vi "Read.vi"(7 "timeout (100ms)":i32=100, 8 "error in (no error)":errorcluster, 9 "Interlock in":bool, 11 "Interlock in":refnum<class "Interlock.lvclass">) -> (0 "error out":errorcluster, 1 "Interlock out":bool, 2 "Data out":variant, 3 "Interlock out":refnum<class "Interlock.lvclass">, 4 "IL Action":refnum<class "IL Action.lvclass">[](array[class]))   [LabVIEW 2015, in "Interlocks.lvlib" / "Interlock.lvclass"]
uses:
  Interlock.lvclass
  IL Action/IL Action.lvclass
  Interlock.lvclass/Interlock.ctl
  State Enum.ctl
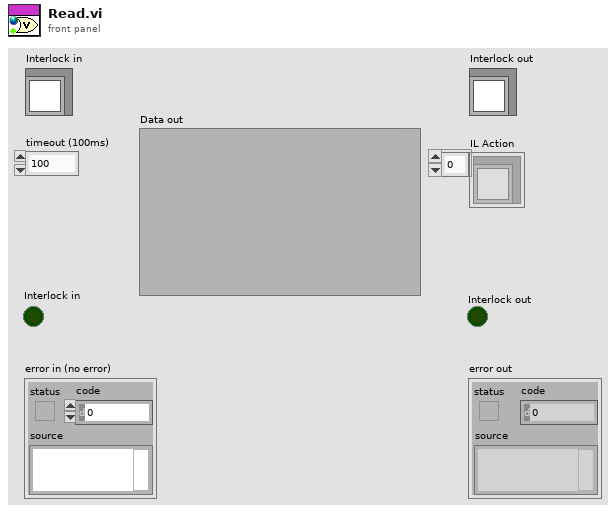
[diagram p1: front panel]
types:
  T1 = typedef "Interlocks.lvlib/Interlock.lvclass/State Enum.ctl" = enum16{"Ok", "Error", "Interlock", "Out of Range", "Is ON", "Is OFF", "Denied", "Not Allowed", "Sample Allow", "Sample Deny"}
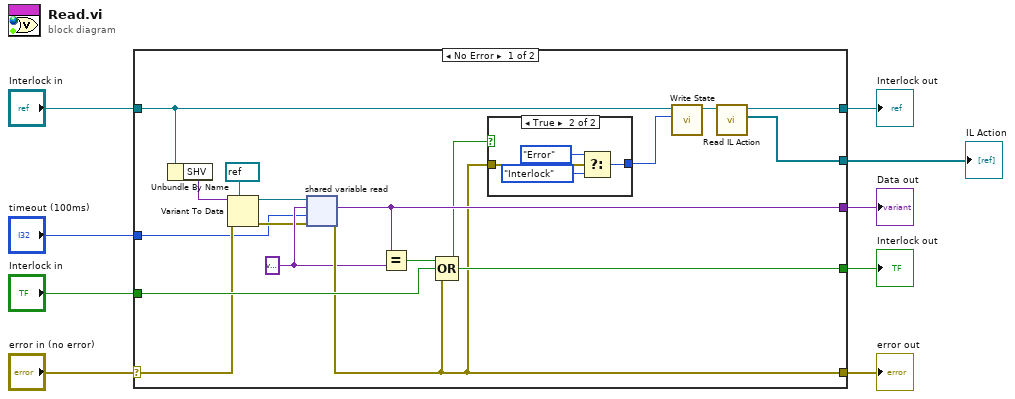
[diagram p0: block diagram]
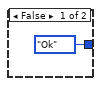
[diagram p2: hidden frame]
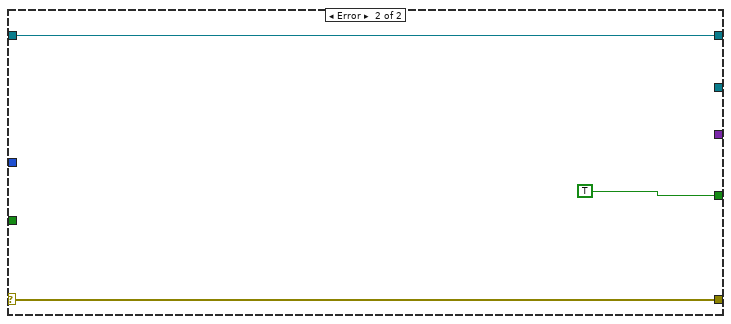
[diagram p3: hidden frame]
diagram:
  n1 = case shown="No Error" "error in (no error)" {
    selector: "error in (no error)" -> [w18 w34]
    tunnel: [w22 w34] -> w8
    tunnel: [w12 w33] -> w6
    tunnel: "Interlock in" -> [w21 w33]
    tunnel: [w26 _] -> w5
    tunnel: [w23 TRUE] -> w4
    tunnel: "Interlock in" -> [w24 _]
    tunnel: "timeout (100ms)" -> [w10 _]
    tunnel: [w11 _] -> w1
    frame No Error {
      w19 = variant ("variant")
      n2 = Unbundle By Name(w21) -> ("SHV"=w16:variant)
      n3 = Variant To Data(error in=w18, type=refnum<k21> refnum ("shared variable refnum in"), Variant=w16) -> (data=w14:refnum<k21>, error out=w17:errorcluster)
      n4 = shared-variable-read(w14, w17, w19, w10) -> (w22:errorcluster, w26:variant)  [unwired: 3 out]
      n5 = Equal?(x=w26, y=w19) -> (x = y?=w25:bool)
      n6 = Compound Arithmetic op=OR(w25, w24, w22) -> (w23:bool)
      n7 = case shown="True" w23 {
        tunnel: w22 -> [_ w31]
        tunnel: [State_Enum."Ok" ("State") w28] -> w20
        frame False {
        }
        frame True {
          n8 = Select(t=State_Enum."Error", s=w31, f=State_Enum."Interlock" ("State")) -> (s? t:f=w28:T1)
        }
      }
      n9 = call "Write State.vi"("State"=w20, "Interlock in"=w21) -> ("Interlock out"=w13:refnum<class "Interlock.lvclass">)  [unwired: 9 in]
      n10 = call "Read IL Action.vi"("Interlock in"=w13) -> ("IL Action"=w11:refnum<class "IL Action.lvclass">[], "Interlock out"=w12:refnum<class "Interlock.lvclass">)  [unwired: 9 in]
    }
    frame Error {
    }
  }
  "error out" <- w8
  "Interlock out" <- w6
  "Data out" <- w5
  "Interlock out" <- w4
  "IL Action" <- w1
